vi "read SQL columns.vi"() -> ()   [LabVIEW 2017]
uses:
  <vilib>/addons/database/Auxilliary.llb/DB Tools DataTypes.ctl
  <vilib>/addons/database/Connection.llb/DB Tools Open Connec (Path).vi
  <vilib>/addons/database/NI_Database_API.lvlib
panel:
  out "cluster":T1
  out "column information":T3(array[cluster])
  out "columns":string[](array[string])
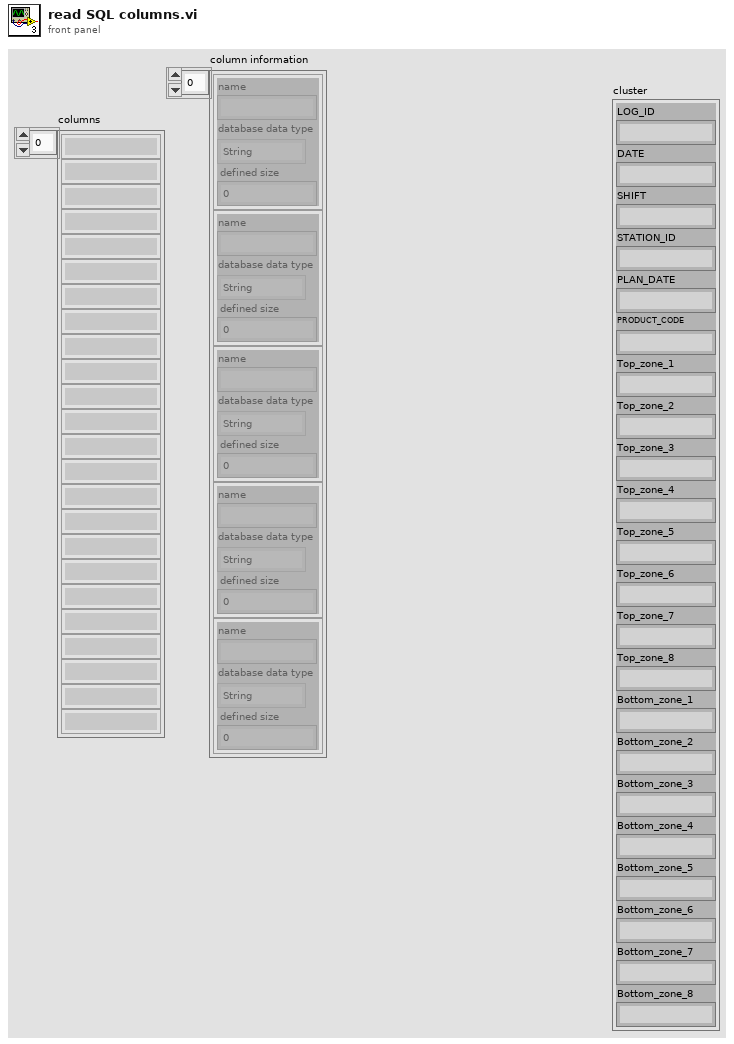
[diagram p1: front panel]
types:
  T1 = cluster{"LOG_ID":string, "DATE":string, "SHIFT":string, "STATION_ID":string, "PLAN_DATE":string, "PRODUCT_CODE":string, "Top_zone_1":string, "Top_zone_2":string, "Top_zone_3":string, "Top_zone_4":string, "Top_zone_5":string, "Top_zone_6":string, "Top_zone_7":string, "Top_zone_8":string, "Bottom_zone_1":string, "Bottom_zone_2":string, "Bottom_zone_3":string, "Bottom_zone_4":string, "Bottom_zone_5":string, "Bottom_zone_6":string, "Bottom_zone_7":string, "Bottom_zone_8":string}
  T2 = typedef "NI_Database_API.lvlib/DB Tools DataTypes.ctl" = enum16{"String", "Long (I32)", "Single (SGL)", "Double (DBL)", "Date/Time", "Binary"}
  T3 = cluster{"name":string, "database data type":T2, "defined size":i32}[]
  T4 = typedef "NI_Database_API.lvlib/Conn ObjectReference.ctl" = refnum<k1>
  T5 = cluster{"columns[0]":string, "columns[1]":string, "columns[2]":string, "columns[3]":string, "columns[4]":string, "columns[5]":string, "columns[6]":string, "columns[7]":string, "columns[8]":string, "columns[9]":string, "columns[10]":string, "columns[11]":string, "columns[12]":string, "columns[13]":string, "columns[14]":string, "columns[15]":string, "columns[16]":string, "columns[17]":string, "columns[18]":string, "columns[19]":string, "columns[20]":string, "columns[21]":string}
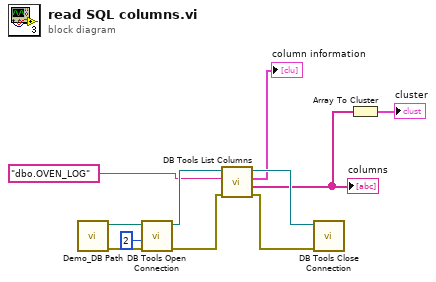
[diagram p0: block diagram]
diagram:
  n1 = call "Demo_DB Path.vi"() -> ("error out"=w10:errorcluster, "DB Path"=w11:path)  [unwired: 10 in]
  n2 = call-poly <vilib>:"DB Tools Open Connection.vi"("error in (no error)"=w10, "connection timeout (15)"=2, "connection information"=w11) -> ("error out"=w8:errorcluster, "connection reference"=w5:T4)  [unwired: 5 in]
  n3 = call <vilib>:"DB Tools List Columns.vi"("error in (no error)"=w8, "table"="dbo.OVEN_LOG", "connection reference"=w5) -> ("error out"=w7:errorcluster, "columns"=w2:string[], "column information"=→"column information":T3, "connection reference out"=w6:T4)  [unwired: 1 in]
  "columns" <- w2
  n4 = call <vilib>:"DB Tools Close Connection.vi"("error in (no error)"=w7, "connection reference"=w6) -> ()  [unwired: 5 in, 1 out]
  n5 = Array To Cluster(array=w2) -> (cluster=→"cluster":T5)
